vi "Scripting_Server_Global.vi"() -> ()   [LabVIEW 2015]
panel:
  out "TCPServer Online":bool
  in  "Port":u16=30050
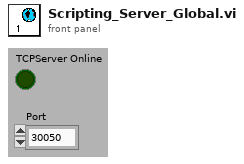
[diagram p1: front panel]
diagram:
